vi "ClassVI.vi"(8 "String2":string="only VIs", 11 "String1":string="Source ") -> (3 "String Output":string)   [LabVIEW 2023, in "Class.lvclass"]
doc: "Output = String1+String2"
uses:
  Class.lvclass
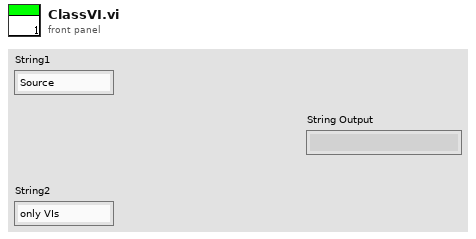
[diagram p1: front panel]
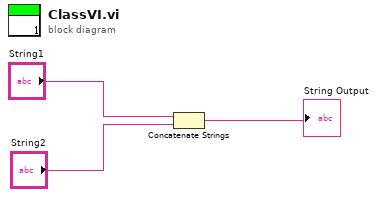
[diagram p0: block diagram]
diagram:
  n1 = Concatenate Strings("String1", "String2") -> (→"String Output":string)
